vi "Write A Theme is Loaded.vi"(8 "error in (no error)":errorcluster, 10 "A Theme is Loaded":bool, 11 "Generic Theme in":refnum<class "Generic Theme.lvclass">) -> (0 "error out":errorcluster, 3 "Generic Theme out":refnum<class "Generic Theme.lvclass">)   [LabVIEW 2021, in "Appearance Actor.lvlib" / "Generic Theme.lvclass"]
doc: "Set whether or not a theme has been loaded from disk (not applied on controls)."
uses:
  Generic Theme.lvclass
  Generic Theme.lvclass/Generic Theme.ctl
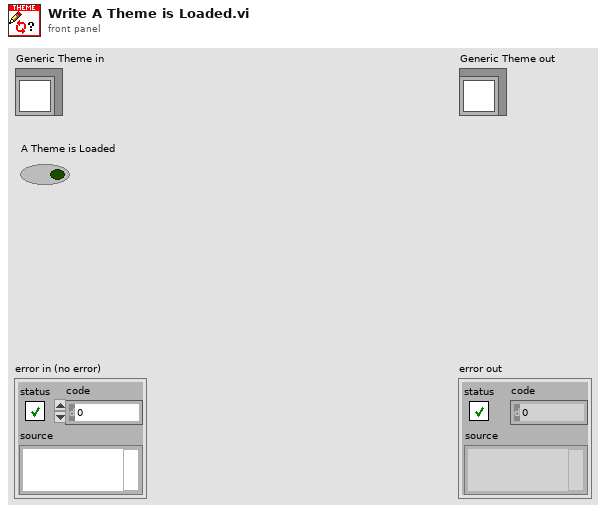
[diagram p1: front panel]
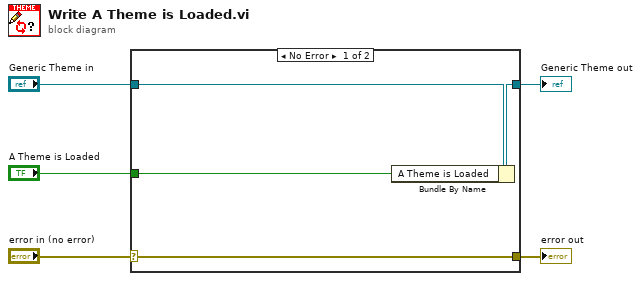
[diagram p0: block diagram]
diagram:
  n1 = case shown="No Error" "error in (no error)" {
    selector: "error in (no error)" -> [w9 w10]
    tunnel: [w9 w10] -> w4
    tunnel: [w7 w11] -> w2
    tunnel: "Generic Theme in" -> [w8 w11]
    tunnel: "A Theme is Loaded" -> [w6 _]
    frame No Error {
      n2 = Bundle By Name(cluster=w8, "A Theme is Loaded"=w6) -> (w7:refnum<class "Generic Theme.lvclass">)
    }
    frame Error {
    }
  }
  "error out" <- w4
  "Generic Theme out" <- w2
